vi "use this to edit build vi.vi"   [LabVIEW 2010]
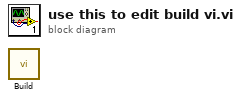
[diagram p0: block diagram]
diagram:
  n1 = call "Build.vi"() -> ()  [unwired: 12 in]
